vi "Replace FP Indicator.vi"(8 "error in (no error)":errorcluster, 11 "Getter Generator In":refnum<class "Getter Generator.lvclass">) -> (0 "error out":errorcluster, 3 "Getter Generator Out":refnum<class "Getter Generator.lvclass">)   [LabVIEW 2020, in "Method Generation.lvlib" / "Getter Generator.lvclass"]
uses:
  Getter Generator.lvclass
  <vilib>/Utility/traverseref.llb/TRef TravTarget.ctl
  Getter Generator.lvclass/Getter Generator.ctl
  <vilib>/Utility/traverseref.llb/VI Scripting - Traverse.lvlib
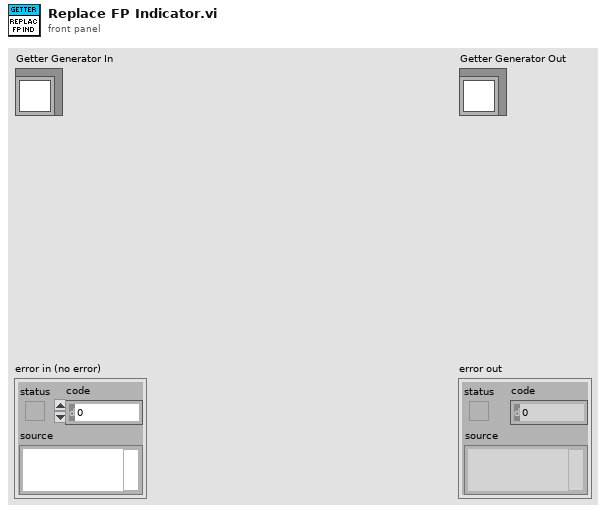
[diagram p1: front panel]
types:
  T1 = typedef "TRef TravTarget.ctl" = enum16{"FP", "BD", "Other"}
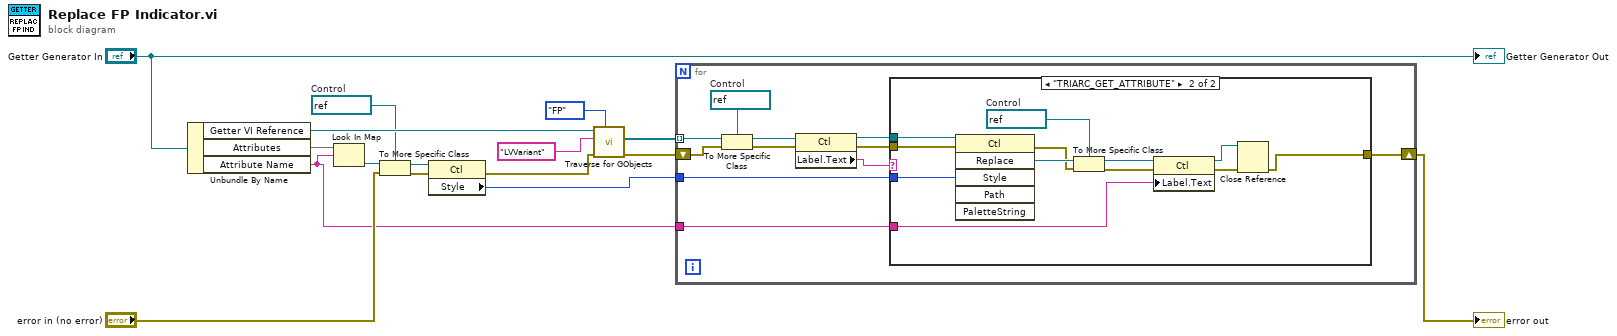
[diagram p0: block diagram]
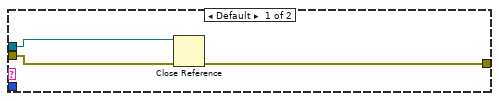
[diagram p2: hidden frame]
diagram:
  w8 = refnum<vi> refnum  # Control
  n1 = Unbundle By Name("Getter Generator In") -> ("Getter VI Reference"=w15:refnum<vi>, "Attributes"=w11:map{string, refnum<vi>}, "Attribute Name"=w1:string)
  n2 = Look In Map(map=w11, key=w1) -> (value=w10:refnum<vi>)  [unwired: 1 in, 1 out]
  n3 = To More Specific Class(target class=w8, reference=w10, error in="error in (no error)") -> (specific class reference=w9:refnum<vi>, error out=w6:errorcluster)
  n4 = property class="Ctl"(reference=w9, error in=w6) -> (error out=w4:errorcluster, "Style"=w7:u32)  [unwired: 1 out]
  n5 = call <vilib>:"Traverse for GObjects.vi"("Traverse Target"=TRef_TravTarget."FP", "error in (no error)"=w4, "Class Name"="LVVariant", "VI Refnum"=w15) -> ("error out"=w12:errorcluster, "References"=w13:refnum<vi>[])  [unwired: 4 in, 2 out]
  n6 = for {
    tunnel: w13 -> [w27] mode=indexing
    tunnel: w7 -> [w24]
    shift-right: [w22] -> w3
    shift-left: w12 -> [w25]
    tunnel: w1 -> [w17]
    w26 = refnum<vi> refnum  # Control
    n7 = To More Specific Class(target class=w26, reference=w27, error in=w25) -> (specific class reference=w20:refnum<vi>, error out=w23:errorcluster)
    n8 = property class="Ctl"(reference=w20, error in=w23) -> (reference out=w19:refnum<vi>, error out=w21:errorcluster, "Label.Text"=w18:string)
    n9 = case shown="\"TRIARC_GET_ATTRIBUTE\"" w18 {
      tunnel: w24 -> [_ w42]
      tunnel: [w29 w31] -> w22
      tunnel: w21 -> [w30 w41]
      tunnel: w19 -> [w28 w40]
      tunnel: w17 -> [_ w34]
      frame Default {
        n10 = Close Reference(reference=w28, error in (no error)=w30) -> (error out=w29:errorcluster)
      }
      frame "TRIARC_GET_ATTRIBUTE" {
        w37 = refnum<vi> refnum  # Control
        n11 = invoke class="Ctl" method="Replace"(reference=w40, error in=w41, "Style"=w42) -> (error out=w36:errorcluster, "Replace"=w39:refnum<vi>)  [unwired: 3 in, 4 out]
        n12 = To More Specific Class(target class=w37, reference=w39, error in=w36) -> (specific class reference=w38:refnum<vi>, error out=w35:errorcluster)
        n13 = property class="Ctl"(reference=w38, error in=w35, "Label.Text"=w34) -> (reference out=w32:refnum<vi>, error out=w33:errorcluster)
        n14 = Close Reference(reference=w32, error in (no error)=w33) -> (error out=w31:errorcluster)
      }
    }
  }
  "error out" <- w3
  "Getter Generator Out" <- "Getter Generator In"
